vi "OFDM_FrequencyOffsetEstimation(CP).vi"(10 "sampling period":dbl format="%#_13g", 11 "input OFDM symbol":cdb[](array[numeric])) -> (3 "output OFDM symbol":cdb[](array[numeric]))   [LabVIEW 2022 SP3]
uses:
  <vilib>/Analysis/baseanly.llb/Mean (DBL).vi
  <vilib>/Analysis/NI_AALBase.lvlib
panel:
  out "frequency offset(CP)":dbl
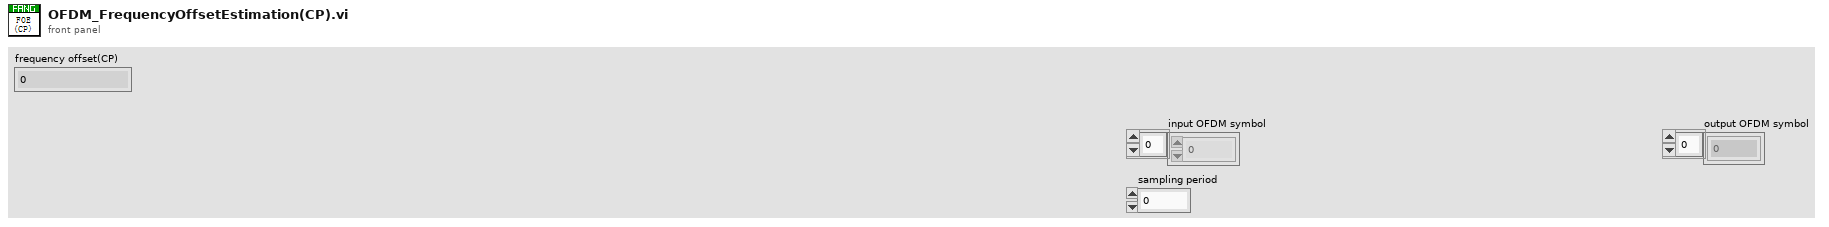
[diagram p1: front panel]
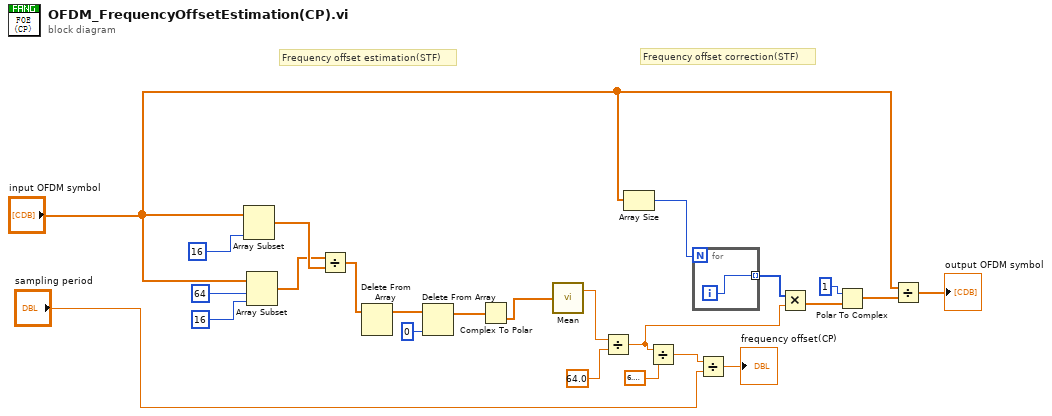
[diagram p0: block diagram]
diagram:
  # "Frequency offset correction(STF)"
  # "Frequency offset estimation(STF)"
  n1 = Array Subset(array="input OFDM symbol", length=16) -> (w9:cdb[])  [unwired: 1 in]
  n2 = Array Subset(array="input OFDM symbol", index=64, length=16) -> (w8:cdb[])
  n3 = Divide(x=w8, y=w9) -> (x/y=w10:cdb[])
  n4 = Delete From Array(array=w10) -> (array with subset deleted=w11:cdb[])  [unwired: 2 in, 1 out]
  n5 = Delete From Array(array=w11, index=0) -> (array with subset deleted=w7:cdb[])  [unwired: 1 in, 1 out]
  n6 = Complex To Polar(r * e^(i*theta)=w7) -> (theta=w6:dbl[])  [unwired: 1 out]
  n7 = call-poly <vilib>:"Mean.vi"("X"=w6) -> ("mean"=w16:dbl)  [unwired: 1 out]
  n8 = Divide(x=w16, y=64.0) -> (x/y=w24:dbl)
  n9 = Array Size(array="input OFDM symbol") -> (size(s)=w2:i32)
  n10 = Divide(x=w24, y=6.283185307179586) -> (x/y=w18:dbl)
  n11 = for {
    N: w2 -> [_]
    tunnel: [w25] -> w1 mode=indexing
    i -> [w25]
  }
  n12 = Divide(x=w18, y="sampling period") -> (x/y=→"frequency offset(CP)":dbl)
  n13 = Multiply(x=w1, y=w24) -> (x*y=w5:dbl[])
  n14 = Polar To Complex(1:w5, 2:1) -> (0:w4:cdb[])
  n15 = Divide(x="input OFDM symbol", y=w4) -> (x/y=→"output OFDM symbol":cdb[])
